vi "RichToFlatni_bus_monitor_api_PassThruReply.vi"(5 "OutputClusterType":T1, 11 "InputCluster":T3) -> (3 "OutputCluster":T1)   [LabVIEW 2025, in "bus_monitor_client.lvlib"]
uses:
  ni_bus_monitor_api_PassThruReply.ctl
  ni_bus_monitor_api_ErrorInfo.ctl
  ni_bus_monitor_api_PassThruReply_Flat.ctl
  ni_bus_monitor_api_ErrorInfo_Flat.ctl
  bus_monitor_client.lvlib
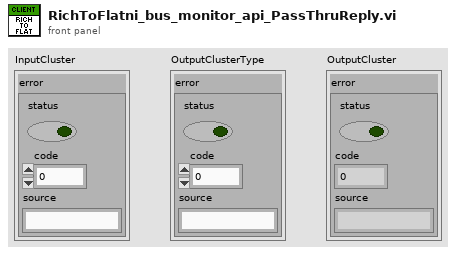
[diagram p1: front panel]
types:
  T1 = typedef "bus_monitor_client.lvlib/ni_bus_monitor_api_PassThruReply_Flat.ctl" = cluster{"error":T2}
  T2 = typedef "bus_monitor_client.lvlib/ni_bus_monitor_api_ErrorInfo_Flat.ctl" = errorcluster
  T3 = typedef "bus_monitor_client.lvlib/ni_bus_monitor_api_PassThruReply.ctl" = cluster{"error":T4}
  T4 = typedef "bus_monitor_client.lvlib/ni_bus_monitor_api_ErrorInfo.ctl" = errorcluster
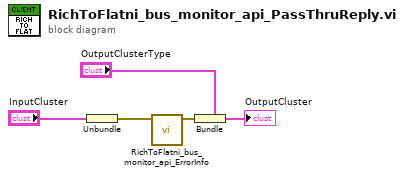
[diagram p0: block diagram]
diagram:
  n1 = Unbundle "Unbundle"("InputCluster") -> ("error"=w2:T4)
  n2 = call "RichToFlatni_bus_monitor_api_ErrorInfo.vi"("InputCluster"=w2) -> ("OutputCluster"=w1:T2)  [unwired: 10 in]
  n3 = Bundle "Bundle"(cluster="OutputClusterType", "error"=w1) -> (→"OutputCluster":T1)
